vi "myRIO_BRig_RT_dataExp_CueLed_Tpeak.vi"() -> (2 "output_CueLed_Tpeak":i32)   [LabVIEW 2014]
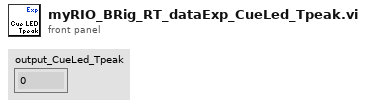
[diagram p1: front panel]
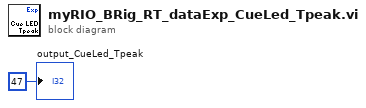
[diagram p0: block diagram]
diagram:
  "output_CueLed_Tpeak" <- 47 ("output_iBlock")
